vi "display.vi"(8 "error in (no error)":errorcluster, 11 "Waveform Graph 2":dynamicdata(graph)) -> (0 "error out":errorcluster, 3 "Waveform Graph":dynamicdata(graph))   [LabVIEW 2021]
doc: "本VI是为《我和LabVIEW》一书编写的示例。\n关于本书的介绍请参考网页：\nhttp://ruanqizhen.spaces.live.com/blog/cns!5852D4F797C53FB6!4310.entry"
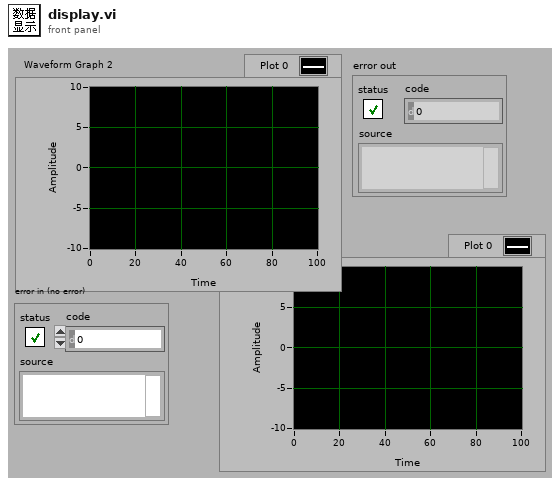
[diagram p1: front panel]
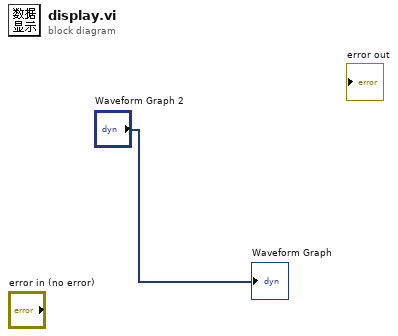
[diagram p0: block diagram]
diagram:
  "Waveform Graph" <- "Waveform Graph 2"
